vi "Motor Manager.vi"() -> ()   [LabVIEW 2014]
uses:
  Typedef/States - PC.ctl
  Typedef/Management variables.ctl
  LV Library/Typedef/Move type.ctl
  <vilib>/Instr/_visa.llb/VISA Configure Serial Port (Instr).vi
  LV Library/Motor manager.lvlib
panel:
  in  "Tab":enum32{"Manual movement", "Cycle"}(tab)
  in  "Down Button":bool
  in  "Up Button":bool
  in  "Right Button":bool
  in  "Left Button":bool
  in  "Speed":cluster{"Speed X":sgl, "Speed Y":sgl}={"Speed X"=10.0, "Speed Y"=10.0}
  in  "Acceleration":T1={"Acceleration X"=10, "Acceleration Y"=10}
  in  "Move type":enum32{"Absolute", "Step", "Free"}(radio)
  in  "Step":cluster{"Step X":sgl, "Step Y":sgl}={"Step X"=200.0, "Step Y"=200.0}
  in  "Cycle settings":T2
  in  "Stop process":bool
  in  "Keep torque":bool
  in  "Make Home":bool
  in  "Find Home":bool
  out "Connected?":bool
  in  "Connect":bool
  in  "VISA in":refnum<visa-resource-name>
  in  "Exit":bool
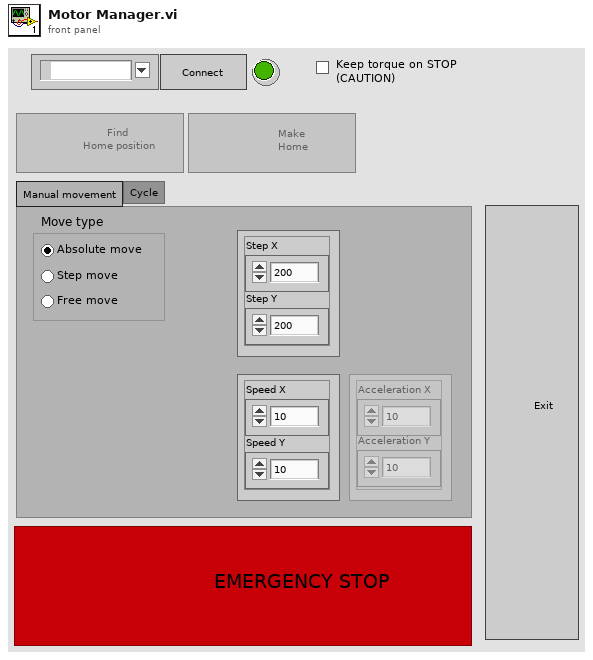
[diagram p1: front panel]
types:
  T1 = cluster{"Acceleration X":i32, "Acceleration Y":i32}
  T2 = cluster{"Motor":u8, "Distance":i32, "Speed":sgl, "IM delay":i32, "Cycle type":enum16{"Move forward first", "Move backward first"}, "N cycles":i32, "Go cycle":bool}
  T3 = typedef "Management variables.ctl" = cluster{"Keep torque":bool}
  T4 = typedef "States - PC.ctl" = enum16{"Connect", "Set speed", "Set management var", "Find Home", "Make Home", "Free Move up", "Free Move down", "Free Move right", "Free Move left", "Stop", "Step Move up", "Step Move down", "Step Move right", "Step Move left", "Simple Cycle", "Stop process", "Exit"}
  T5 = typedef "Motor manager.lvlib/Move type.ctl" = enum16{"Move forward", "Move backward", "Cycle (forward first)", "Cycle (backward first)", "Move step forward", "Move step backward"}
  T6 = cluster{T4, "Step":cluster{"Step X":sgl, "Step Y":sgl}}
  T7 = cluster{T4, "Cycle settings":cluster{"Motor":u8, "Distance":i32, "Speed":sgl, "IM delay":i32, "Cycle type":enum16{"Move forward first", "Move backward first"}, "N cycles":i32, "Go cycle":bool}}
  T8 = cluster{T4, "Speed":cluster{"Speed X":sgl, "Speed Y":sgl}}
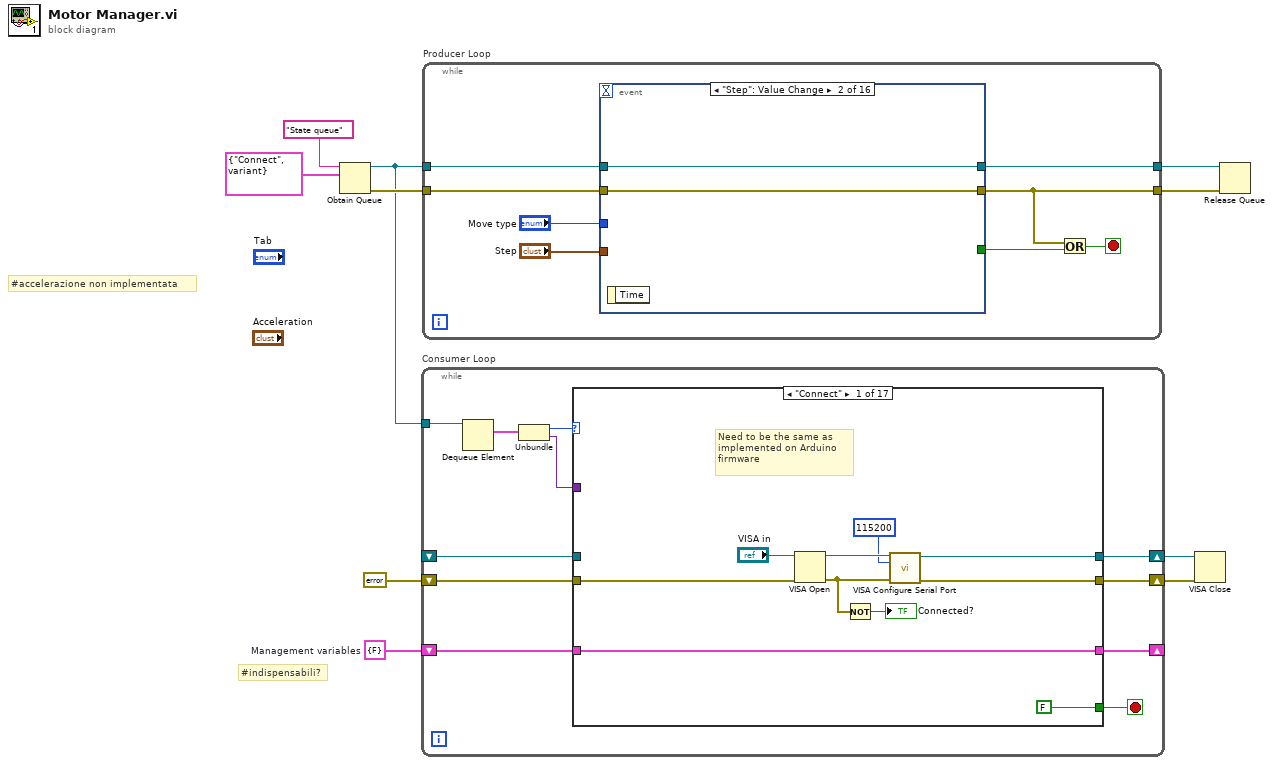
[diagram p0: block diagram]
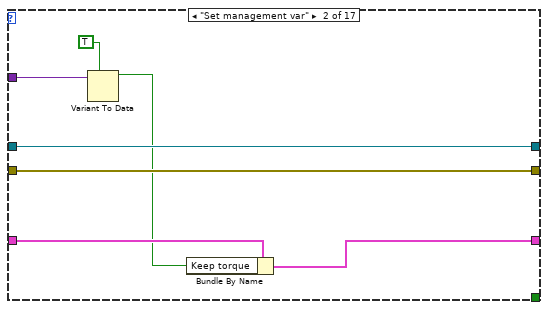
[diagram p2: hidden frame]
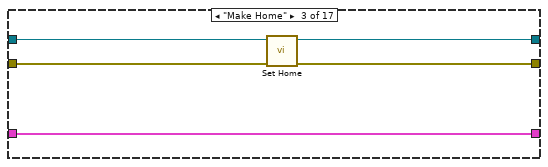
[diagram p3: hidden frame]
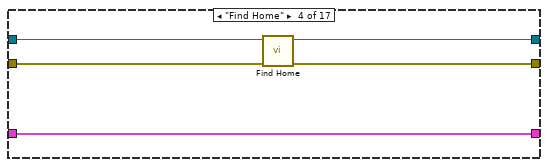
[diagram p4: hidden frame]
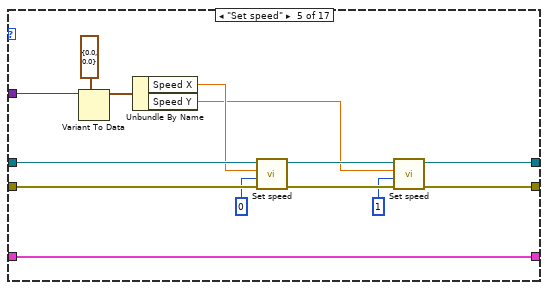
[diagram p5: hidden frame]
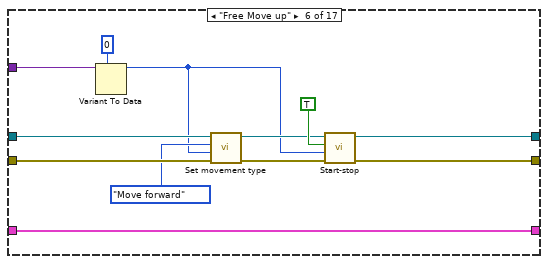
[diagram p6: hidden frame]
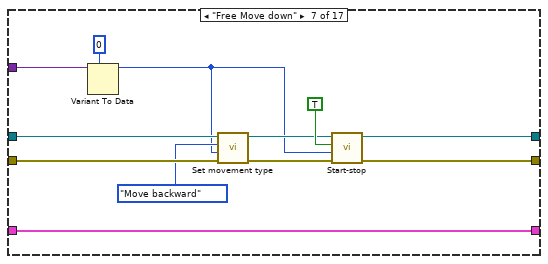
[diagram p7: hidden frame]
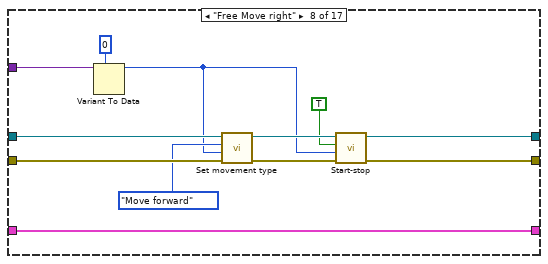
[diagram p8: hidden frame]
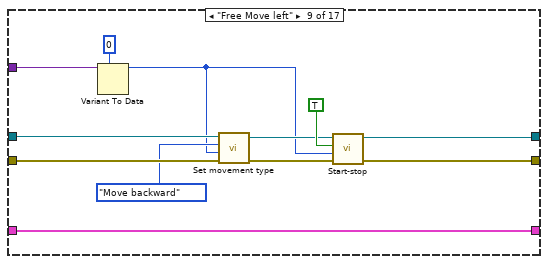
[diagram p9: hidden frame]
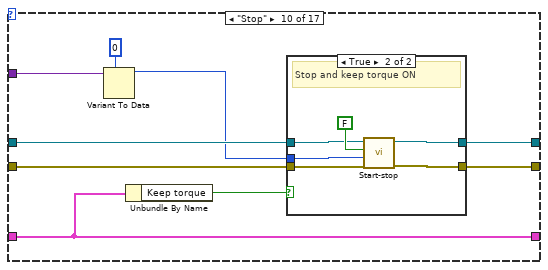
[diagram p10: hidden frame]
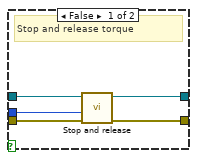
[diagram p11: hidden frame]
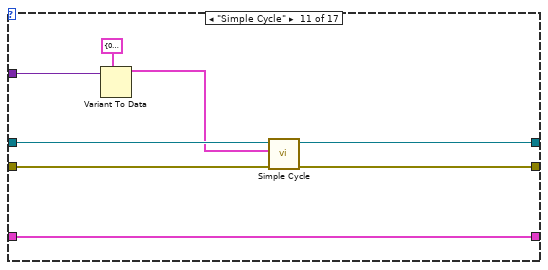
[diagram p12: hidden frame]
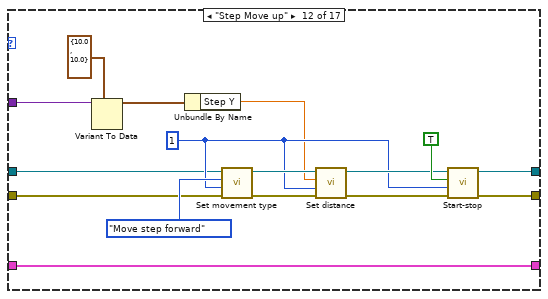
[diagram p13: hidden frame]
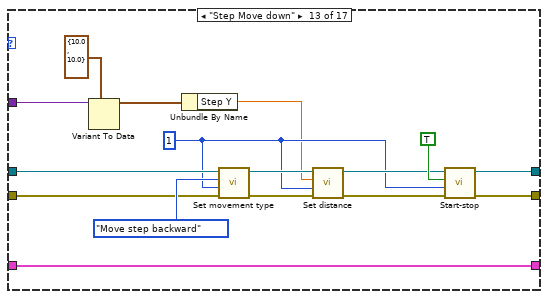
[diagram p14: hidden frame]
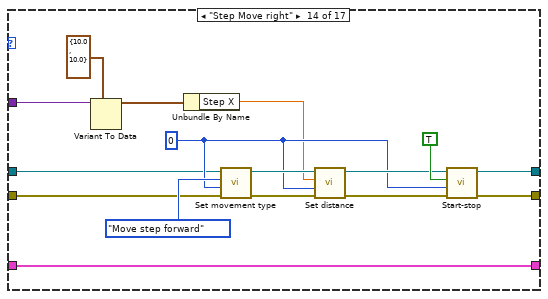
[diagram p15: hidden frame]
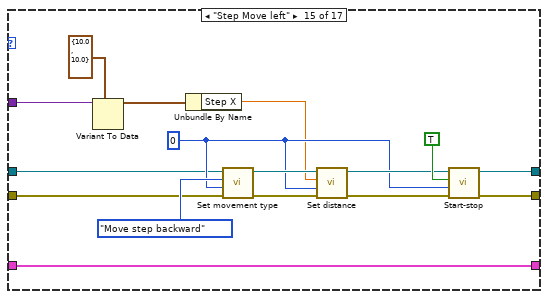
[diagram p16: hidden frame]
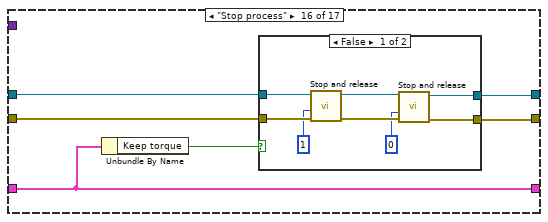
[diagram p17: hidden frame]
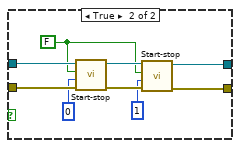
[diagram p18: hidden frame]
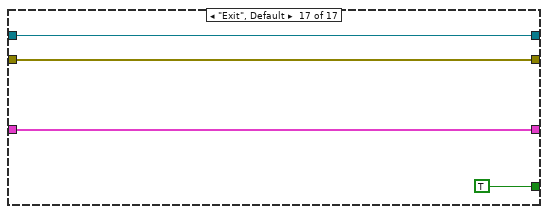
[diagram p19: hidden frame]
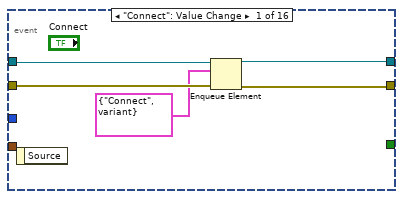
[diagram p20: hidden frame]
diagram:
  w2 = T3 {"Keep torque"=FALSE}  # Management variables
  # "#accelerazione non implementata"
  # "#indispensabili?"
  n1 = Obtain Queue(name (unnamed)="State queue", element data type=cluster{T4, variant} {enum."Connect", variant}) -> (queue out=w6:refnum<queue>, error out=w10:errorcluster)  [unwired: 3 in, 1 out]
  n2 = while "Consumer Loop" {
    tunnel: w6 -> [w21]
    shift-right: [w19] -> w5
    shift-left: _ -> [w17]
    shift-right: [w18] -> w4
    shift-left: errorcluster {"status"=FALSE, "code"=0, "source"=""} ("Error Out") -> [w16]
    shift-right: [w11] -> _
    shift-left: w2 -> [w12]
    stop <- w20 stop-if-true
    n3 = Dequeue Element(queue=w21) -> (element=w15:cluster{T4, variant})  [unwired: 2 in, 3 out]
    n4 = Unbundle(w15) -> (w14:T4, w13:variant)
    n5 = case shown="\"Connect\"" w14 {
      tunnel: [FALSE _ _ _ _ _ _ _ _ _ _ _ _ _ _ _ TRUE] -> w20
      tunnel: [w27 w38 w41 w45 w59 w73 w81 w93 w105 w118 w136 w140 w163 w173 w189 w206 w227] -> w19
      tunnel: [w26 w37 w39 w44 w60 w72 w80 w92 w104 w119 w135 w141 w164 w172 w188 w205 w226] -> w18
      tunnel: w17 -> [_ w38 w42 w46 w57 w70 w83 w94 w106 w117 w137 w143 w167 w175 w191 w208 w227]
      tunnel: w16 -> [w25 w37 w40 w47 w62 w71 w82 w95 w107 w116 w134 w142 w166 w176 w190 w207 w226]
      tunnel: w13 -> [_ w36 _ _ w56 w65 w78 w89 w101 w115 w132 w144 w168 w174 w192 _ _]
      tunnel: w12 -> [w22 w34 w43 w48 w49 w63 w75 w87 w99 w111 w138 w139 w165 w171 w187 w203 w228]
      tunnel: [w22 w32 w43 w48 w49 w63 w75 w87 w99 w111 w138 w139 w165 w171 w187 w203 w228] -> w11
      frame "Connect" {
        # "Need to be the same as \nimplemented on Arduino\nfirmware"
        n6 = VISA Open(error in (no error)=w25, VISA resource name="VISA in") -> (VISA resource name=w29:refnum<visa-resource-name>, error out=w24:errorcluster)  [unwired: 3 in]
        n7 = Not(x=w24) -> (.not. x?=→"Connected?":bool)
        n8 = call-poly "VISA Configure Serial Port"("VISA resource name"=w29, "baud rate (9600)"=u32 115200, "error in (no error)"=w24) -> ("VISA resource name out"=w27:refnum<visa-resource-name>, "error out"=w26:errorcluster)  [unwired: 11 in]
      }
      frame "Set management var" {
        n9 = Variant To Data(type=TRUE, Variant=w36) -> (data=w33:bool)  [unwired: 1 in, 1 out]
        n10 = Bundle By Name(cluster=w34, "Keep torque"=w33) -> (w32:T3)
      }
      frame "Make Home" {
        n11 = call "Set Home.vi"("Error In"=w40, "VISA resource in"=w42) -> ("Error Out"=w39:errorcluster, "VISA resource out"=w41:refnum<visa-resource-name>)  [unwired: 8 in]
      }
      frame "Find Home" {
        n12 = call "Find Home.vi"("Error In"=w47, "VISA resource in"=w46) -> ("Error Out"=w44:errorcluster, "VISA resource out"=w45:refnum<visa-resource-name>)  [unwired: 8 in]
      }
      frame "Set speed" {
        n13 = Variant To Data(type=cluster{"Speed X":sgl, "Speed Y":sgl} {"Speed X"=0.0, "Speed Y"=0.0} ("Speed 2"), Variant=w56) -> (data=w54:cluster{"Speed X":sgl, "Speed Y":sgl})  [unwired: 1 in, 1 out]
        n14 = Unbundle By Name(w54) -> ("Speed X"=w53:sgl, "Speed Y"=w52:sgl)
        n15 = call "Set speed.vi"("Error In"=w62, "Motor index"=u8 0, "Speed"=w53, "VISA resource in"=w57) -> ("Error Out"=w61:errorcluster, "VISA resource out"=w58:refnum<visa-resource-name>)  [unwired: 6 in]
        n16 = call "Set speed.vi"("Error In"=w61, "Motor index"=u8 1, "Speed"=w52, "VISA resource in"=w58) -> ("Error Out"=w60:errorcluster, "VISA resource out"=w59:refnum<visa-resource-name>)  [unwired: 6 in]
      }
      frame "Free Move up" {
        n17 = Variant To Data(type=u8 0, Variant=w65) -> (data=w64:u8)  [unwired: 1 in, 1 out]
        n18 = call "Set movement type.vi"("Error In"=w71, "Motor index"=w64, "Movement type"=Move_type."Move forward", "VISA resource in"=w70) -> ("Error Out"=w69:errorcluster, "VISA resource out"=w68:refnum<visa-resource-name>)  [unwired: 6 in]
        n19 = call "Start-stop.vi"("Error In"=w69, "Motor index"=w64, "Go"=TRUE, "VISA resource in"=w68) -> ("Error Out"=w72:errorcluster, "VISA resource out"=w73:refnum<visa-resource-name>)  [unwired: 6 in]
      }
      frame "Free Move down" {
        n20 = Variant To Data(type=u8 0, Variant=w78) -> (data=w76:u8)  [unwired: 1 in, 1 out]
        n21 = call "Set movement type.vi"("Error In"=w82, "Motor index"=w76, "Movement type"=Move_type."Move backward", "VISA resource in"=w83) -> ("Error Out"=w85:errorcluster, "VISA resource out"=w84:refnum<visa-resource-name>)  [unwired: 6 in]
        n22 = call "Start-stop.vi"("Error In"=w85, "Motor index"=w76, "Go"=TRUE, "VISA resource in"=w84) -> ("Error Out"=w80:errorcluster, "VISA resource out"=w81:refnum<visa-resource-name>)  [unwired: 6 in]
      }
      frame "Free Move right" {
        n23 = Variant To Data(type=u8 0, Variant=w89) -> (data=w88:u8)  [unwired: 1 in, 1 out]
        n24 = call "Set movement type.vi"("Error In"=w95, "Motor index"=w88, "Movement type"=Move_type."Move forward", "VISA resource in"=w94) -> ("Error Out"=w97:errorcluster, "VISA resource out"=w98:refnum<visa-resource-name>)  [unwired: 6 in]
        n25 = call "Start-stop.vi"("Error In"=w97, "Motor index"=w88, "Go"=TRUE, "VISA resource in"=w98) -> ("Error Out"=w92:errorcluster, "VISA resource out"=w93:refnum<visa-resource-name>)  [unwired: 6 in]
      }
      frame "Free Move left" {
        n26 = Variant To Data(type=u8 0, Variant=w101) -> (data=w100:u8)  [unwired: 1 in, 1 out]
        n27 = call "Set movement type.vi"("Error In"=w107, "Motor index"=w100, "Movement type"=Move_type."Move backward", "VISA resource in"=w106) -> ("Error Out"=w109:errorcluster, "VISA resource out"=w108:refnum<visa-resource-name>)  [unwired: 6 in]
        n28 = call "Start-stop.vi"("Error In"=w109, "Motor index"=w100, "Go"=TRUE, "VISA resource in"=w108) -> ("Error Out"=w104:errorcluster, "VISA resource out"=w105:refnum<visa-resource-name>)  [unwired: 6 in]
      }
      frame "Stop" {
        n29 = Variant To Data(type=u8 0, Variant=w115) -> (data=w113:u8)  [unwired: 1 in, 1 out]
        n30 = Unbundle By Name(w111) -> ("Keep torque"=w112:bool)
        n31 = case shown="True" w112 {
          tunnel: [w120 w129] -> w119
          tunnel: [w123 w128] -> w118
          tunnel: w117 -> [w124 w127]
          tunnel: w116 -> [w122 w126]
          tunnel: w113 -> [w121 w125]
          frame False {
            # "Stop and release torque"
            n32 = call "Stop and release.vi"("Error In"=w122, "Motor index"=w121, "VISA resource in"=w124) -> ("Error Out"=w120:errorcluster, "VISA resource out"=w123:refnum<visa-resource-name>)  [unwired: 7 in]
          }
          frame True {
            # "Stop and keep torque ON"
            n33 = call "Start-stop.vi"("Error In"=w126, "Motor index"=w125, "Go"=FALSE, "VISA resource in"=w127) -> ("Error Out"=w129:errorcluster, "VISA resource out"=w128:refnum<visa-resource-name>)  [unwired: 6 in]
          }
        }
      }
      frame "Simple Cycle" {
        n34 = Variant To Data(type=T2 {"Motor"=0, "Distance"=0, "Speed"=0.0, "IM delay"=0, "Cycle type"=enum."Move forward first", "N cycles"=0, "Go cycle"=FALSE} ("Cycle settings 2"), Variant=w132) -> (data=w131:T2)  [unwired: 1 in, 1 out]
        n35 = call "Simple Cycle.vi"("Error In"=w134, "Cycle settings"=w131, "VISA in"=w137) -> ("Error Out"=w135:errorcluster, "VISA out"=w136:refnum<visa-resource-name>)  [unwired: 7 in]
      }
      frame "Step Move up" {
        w147 = u8 1
        n36 = Variant To Data(type=cluster{"Step X":sgl, "Step Y":sgl} {"Step X"=10.0, "Step Y"=10.0} ("Step"), Variant=w144) -> (data=w146:cluster{"Step X":sgl, "Step Y":sgl})  [unwired: 1 in, 1 out]
        n37 = Unbundle By Name(w146) -> ("Step Y"=w145:sgl)
        n38 = call "Set movement type.vi"("Error In"=w142, "Motor index"=w147, "Movement type"=Move_type."Move step forward", "VISA resource in"=w143) -> ("Error Out"=w151:errorcluster, "VISA resource out"=w152:refnum<visa-resource-name>)  [unwired: 6 in]
        n39 = call "Set distance.vi"("Error In"=w151, "Motor index"=w147, "Travel distance"=w145, "VISA resource in"=w152) -> ("Error Out"=w150:errorcluster, "VISA resource out"=w149:refnum<visa-resource-name>)  [unwired: 6 in]
        n40 = call "Start-stop.vi"("Error In"=w150, "Motor index"=w147, "Go"=TRUE, "VISA resource in"=w149) -> ("Error Out"=w141:errorcluster, "VISA resource out"=w140:refnum<visa-resource-name>)  [unwired: 6 in]
      }
      frame "Step Move down" {
        w157 = u8 1
        n41 = Variant To Data(type=cluster{"Step X":sgl, "Step Y":sgl} {"Step X"=10.0, "Step Y"=10.0} ("Step"), Variant=w168) -> (data=w156:cluster{"Step X":sgl, "Step Y":sgl})  [unwired: 1 in, 1 out]
        n42 = Unbundle By Name(w156) -> ("Step Y"=w155:sgl)
        n43 = call "Set movement type.vi"("Error In"=w166, "Motor index"=w157, "Movement type"=Move_type."Move step backward", "VISA resource in"=w167) -> ("Error Out"=w161:errorcluster, "VISA resource out"=w162:refnum<visa-resource-name>)  [unwired: 6 in]
        n44 = call "Set distance.vi"("Error In"=w161, "Motor index"=w157, "Travel distance"=w155, "VISA resource in"=w162) -> ("Error Out"=w160:errorcluster, "VISA resource out"=w159:refnum<visa-resource-name>)  [unwired: 6 in]
        n45 = call "Start-stop.vi"("Error In"=w160, "Motor index"=w157, "Go"=TRUE, "VISA resource in"=w159) -> ("Error Out"=w164:errorcluster, "VISA resource out"=w163:refnum<visa-resource-name>)  [unwired: 6 in]
      }
      frame "Step Move right" {
        w179 = u8 0
        n46 = Variant To Data(type=cluster{"Step X":sgl, "Step Y":sgl} {"Step X"=10.0, "Step Y"=10.0} ("Step"), Variant=w174) -> (data=w178:cluster{"Step X":sgl, "Step Y":sgl})  [unwired: 1 in, 1 out]
        n47 = Unbundle By Name(w178) -> ("Step X"=w177:sgl)
        n48 = call "Set movement type.vi"("Error In"=w176, "Motor index"=w179, "Movement type"=Move_type."Move step forward", "VISA resource in"=w175) -> ("Error Out"=w183:errorcluster, "VISA resource out"=w184:refnum<visa-resource-name>)  [unwired: 6 in]
        n49 = call "Set distance.vi"("Error In"=w183, "Motor index"=w179, "Travel distance"=w177, "VISA resource in"=w184) -> ("Error Out"=w182:errorcluster, "VISA resource out"=w181:refnum<visa-resource-name>)  [unwired: 6 in]
        n50 = call "Start-stop.vi"("Error In"=w182, "Motor index"=w179, "Go"=TRUE, "VISA resource in"=w181) -> ("Error Out"=w172:errorcluster, "VISA resource out"=w173:refnum<visa-resource-name>)  [unwired: 6 in]
      }
      frame "Step Move left" {
        w195 = u8 0
        n51 = Variant To Data(type=cluster{"Step X":sgl, "Step Y":sgl} {"Step X"=10.0, "Step Y"=10.0} ("Step"), Variant=w192) -> (data=w194:cluster{"Step X":sgl, "Step Y":sgl})  [unwired: 1 in, 1 out]
        n52 = Unbundle By Name(w194) -> ("Step X"=w193:sgl)
        n53 = call "Set movement type.vi"("Error In"=w190, "Motor index"=w195, "Movement type"=Move_type."Move step backward", "VISA resource in"=w191) -> ("Error Out"=w199:errorcluster, "VISA resource out"=w200:refnum<visa-resource-name>)  [unwired: 6 in]
        n54 = call "Set distance.vi"("Error In"=w199, "Motor index"=w195, "Travel distance"=w193, "VISA resource in"=w200) -> ("Error Out"=w198:errorcluster, "VISA resource out"=w197:refnum<visa-resource-name>)  [unwired: 6 in]
        n55 = call "Start-stop.vi"("Error In"=w198, "Motor index"=w195, "Go"=TRUE, "VISA resource in"=w197) -> ("Error Out"=w188:errorcluster, "VISA resource out"=w189:refnum<visa-resource-name>)  [unwired: 6 in]
      }
      frame "Stop process" {
        n56 = Unbundle By Name(w203) -> ("Keep torque"=w204:bool)
        n57 = case shown="False" w204 {
          tunnel: w208 -> [w215 w223]
          tunnel: w207 -> [w216 w222]
          tunnel: [w211 w221] -> w206
          tunnel: [w212 w220] -> w205
          frame False {
            n58 = call "Stop and release.vi"("Error In"=w216, "Motor index"=u8 1, "VISA resource in"=w215) -> ("Error Out"=w213:errorcluster, "VISA resource out"=w214:refnum<visa-resource-name>)  [unwired: 7 in]
            n59 = call "Stop and release.vi"("Error In"=w213, "Motor index"=u8 0, "VISA resource in"=w214) -> ("Error Out"=w212:errorcluster, "VISA resource out"=w211:refnum<visa-resource-name>)  [unwired: 7 in]
          }
          frame True {
            w217 = FALSE ("Go")
            n60 = call "Start-stop.vi"("Error In"=w222, "Motor index"=u8 0, "Go"=w217, "VISA resource in"=w223) -> ("Error Out"=w224:errorcluster, "VISA resource out"=w225:refnum<visa-resource-name>)  [unwired: 6 in]
            n61 = call "Start-stop.vi"("Error In"=w224, "Motor index"=u8 1, "Go"=w217, "VISA resource in"=w225) -> ("Error Out"=w220:errorcluster, "VISA resource out"=w221:refnum<visa-resource-name>)  [unwired: 6 in]
          }
        }
      }
      frame "Exit", Default {
      }
    }
  }
  n62 = while "Producer Loop" {
    tunnel: w6 -> [w237]
    tunnel: w10 -> [w236]
    tunnel: [w232] -> w8
    tunnel: [w235] -> w7
    stop <- w234 stop-if-true
    n63 = event shown="[1] \"Step\": Value Change" {
      selector: _ -> [_ _ _ _ _ _ _ _ _ _ _ _ _ _ _ _]
      dyn-events: _ -> [_ _ _ _ _ _ _ _ _ _ _ _ _ _ _ _]
      timeout: _ -> [_ _ _ _ _ _ _ _ _ _ _ _ _ _ _ _]
      tunnel: w237 -> [w241 w244 w248 w252 w258 w277 w299 w315 w319 w338 w358 w371 w377 w384 w391 w394]
      tunnel: w236 -> [w242 w243 w249 w251 w257 w278 w298 w314 w318 w337 w357 w370 w378 w383 w390 w395]
      tunnel: [w239 w244 w247 w254 w259 w280 w297 w312 w321 w341 w360 w371 w376 w382 w389 w393] -> w235
      tunnel: [w240 w243 w246 w253 w260 w279 w296 w313 w320 w340 w359 w370 w375 w381 w388 w392] -> w232
      tunnel: [_ _ _ _ _ _ _ _ _ _ _ _ _ TRUE _ _] -> w233
      tunnel: "Move type" -> [_ _ _ _ w256 w276 w295 _ w316 w336 w356 _ _ _ _ _]
      tunnel: "Step" -> [_ _ _ _ w255 w275 _ _ w317 w339 _ _ _ _ _ _]
      event "Connect": Value Change {
        n64 = event-data() -> ()  [unwired: 1 in, 1 out]
        n65 = Enqueue Element(queue=w241, element=cluster{T4, variant} {enum."Connect", variant}, error in (no error)=w242) -> (queue out=w239:refnum<queue>, error out=w240:errorcluster)  [unwired: 1 in, 1 out]
      }
      event "Step": Value Change {
        n66 = event-data() -> ()  [unwired: 1 in, 1 out]
      }
      event "Find Home": Value Change {
        n67 = event-data() -> ()  [unwired: 1 in, 1 out]
        n68 = Enqueue Element(queue=w248, element=cluster{T4, variant} {enum."Find Home", variant}, error in (no error)=w249) -> (queue out=w247:refnum<queue>, error out=w246:errorcluster)  [unwired: 1 in, 1 out]
      }
      event "Make Home": Value Change {
        n69 = event-data() -> ()  [unwired: 1 in, 1 out]
        n70 = Enqueue Element(queue=w252, element=cluster{T4, variant} {enum."Make Home", variant}, error in (no error)=w251) -> (queue out=w254:refnum<queue>, error out=w253:errorcluster)  [unwired: 1 in, 1 out]
      }
      event "Up Button": Mouse Down {
        n71 = event-data() -> ()  [unwired: 1 in, 1 out]
        n72 = case shown="\"Free\", Default" w256 {
          tunnel: [w265 w267 w272] -> w259
          tunnel: [w264 w266 w271] -> w260
          tunnel: w257 -> [w263 w266 w274]
          tunnel: w258 -> [w262 w267 w273]
          tunnel: w255 -> [_ _ w269]
          frame "Free", Default {
            n73 = Enqueue Element(queue=w262, element=cluster{T4, i32} {enum."Free Move up", 1}, error in (no error)=w263) -> (queue out=w265:refnum<queue>, error out=w264:errorcluster)  [unwired: 1 in, 1 out]
          }
          frame "Absolute" {
            # "#notImplemented"
          }
          frame "Step" {
            n74 = Bundle(States_-_PC."Step Move up", "Step"=w269) -> (w268:T6)  [unwired: 1 in]
            n75 = Enqueue Element(queue=w273, element=w268, error in (no error)=w274) -> (queue out=w272:refnum<queue>, error out=w271:errorcluster)  [unwired: 1 in, 1 out]
          }
        }
      }
      event "Down Button": Mouse Down {
        n76 = event-data() -> ()  [unwired: 1 in, 1 out]
        n77 = case shown="\"Free\", Default" w276 {
          tunnel: [w285 w287 w292] -> w280
          tunnel: [w284 w286 w291] -> w279
          tunnel: w278 -> [w283 w286 w294]
          tunnel: w277 -> [w282 w287 w293]
          tunnel: w275 -> [_ _ w289]
          frame "Free", Default {
            n78 = Enqueue Element(queue=w282, element=cluster{T4, i32} {enum."Free Move down", 1}, error in (no error)=w283) -> (queue out=w285:refnum<queue>, error out=w284:errorcluster)  [unwired: 1 in, 1 out]
          }
          frame "Absolute" {
            # "#notImplemented"
          }
          frame "Step" {
            n79 = Bundle(States_-_PC."Step Move down", "Step"=w289) -> (w288:T6)  [unwired: 1 in]
            n80 = Enqueue Element(queue=w293, element=w288, error in (no error)=w294) -> (queue out=w292:refnum<queue>, error out=w291:errorcluster)  [unwired: 1 in, 1 out]
          }
        }
      }
      event "Up Button", "Down Button": Mouse Up {
        n81 = event-data() -> ()  [unwired: 1 in, 1 out]
        n82 = case shown="\"Step\"" w295 {
          tunnel: w299 -> [w301 w303 w308]
          tunnel: w298 -> [w300 w302 w307]
          tunnel: [w301 w303 w306] -> w297
          tunnel: [w300 w302 w305] -> w296
          frame "Absolute", Default {
          }
          frame "Step" {
          }
          frame "Free" {
            n83 = Enqueue Element(queue=w308, element=cluster{T4, u8} {enum."Stop", 1}, error in (no error)=w307) -> (queue out=w306:refnum<queue>, error out=w305:errorcluster)  [unwired: 1 in, 1 out]
          }
        }
      }
      event "Cycle settings.Go cycle": Value Change {
        n84 = event-data() -> ()  [unwired: 1 in, 1 out]
        n85 = Bundle(States_-_PC."Simple Cycle", "Cycle settings"="Cycle settings") -> (w309:T7)  [unwired: 1 in]
        n86 = Enqueue Element(queue=w315, element=w309, error in (no error)=w314) -> (queue out=w312:refnum<queue>, error out=w313:errorcluster)  [unwired: 1 in, 1 out]
      }
      event "Right Button": Mouse Down {
        n87 = event-data() -> ()  [unwired: 1 in, 1 out]
        n88 = case shown="\"Free\", Default" w316 {
          tunnel: [w326 w328 w333] -> w321
          tunnel: [w325 w327 w332] -> w320
          tunnel: w318 -> [w324 w327 w335]
          tunnel: w319 -> [w323 w328 w334]
          tunnel: w317 -> [_ _ w330]
          frame "Free", Default {
            n89 = Enqueue Element(queue=w323, element=cluster{T4, i32} {enum."Free Move right", 0}, error in (no error)=w324) -> (queue out=w326:refnum<queue>, error out=w325:errorcluster)  [unwired: 1 in, 1 out]
          }
          frame "Absolute" {
            # "#notImplemented"
          }
          frame "Step" {
            n90 = Bundle(States_-_PC."Step Move right", "Step"=w330) -> (w329:T6)  [unwired: 1 in]
            n91 = Enqueue Element(queue=w334, element=w329, error in (no error)=w335) -> (queue out=w333:refnum<queue>, error out=w332:errorcluster)  [unwired: 1 in, 1 out]
          }
        }
      }
      event "Left Button": Mouse Down {
        n92 = event-data() -> ()  [unwired: 1 in, 1 out]
        n93 = case shown="\"Free\", Default" w336 {
          tunnel: [w346 w348 w353] -> w341
          tunnel: [w345 w347 w352] -> w340
          tunnel: w337 -> [w344 w347 w355]
          tunnel: w338 -> [w343 w348 w354]
          tunnel: w339 -> [_ _ w350]
          frame "Free", Default {
            n94 = Enqueue Element(queue=w343, element=cluster{T4, i32} {enum."Free Move left", 0}, error in (no error)=w344) -> (queue out=w346:refnum<queue>, error out=w345:errorcluster)  [unwired: 1 in, 1 out]
          }
          frame "Absolute" {
            # "#notImplemented"
          }
          frame "Step" {
            n95 = Bundle(States_-_PC."Step Move left", "Step"=w350) -> (w349:T6)  [unwired: 1 in]
            n96 = Enqueue Element(queue=w354, element=w349, error in (no error)=w355) -> (queue out=w353:refnum<queue>, error out=w352:errorcluster)  [unwired: 1 in, 1 out]
          }
        }
      }
      event "Left Button", "Right Button": Mouse Up {
        n97 = event-data() -> ()  [unwired: 1 in, 1 out]
        n98 = case shown="\"Step\"" w356 {
          tunnel: [w362 w364 w369] -> w360
          tunnel: [w361 w363 w368] -> w359
          tunnel: w358 -> [w362 w364 w367]
          tunnel: w357 -> [w361 w363 w366]
          frame "Absolute", Default {
          }
          frame "Step" {
          }
          frame "Free" {
            n99 = Enqueue Element(queue=w367, element=cluster{T4, u8} {enum."Stop", 0}, error in (no error)=w366) -> (queue out=w369:refnum<queue>, error out=w368:errorcluster)  [unwired: 1 in, 1 out]
          }
        }
      }
      event "Move type": Value Change {
        n100 = event-data() -> ()  [unwired: 1 in, 1 out]
      }
      event "Speed": Value Change {
        n101 = event-data() -> ()  [unwired: 1 in, 6 out]
        n102 = Bundle(States_-_PC."Set speed", "Speed"="Speed") -> (w372:T8)  [unwired: 1 in]
        n103 = Enqueue Element(queue=w377, element=w372, error in (no error)=w378) -> (queue out=w376:refnum<queue>, error out=w375:errorcluster)  [unwired: 1 in, 1 out]
      }
      event "Exit": Value Change {
        n104 = event-data() -> ()  [unwired: 1 in, 1 out]
        n105 = Enqueue Element(queue=w384, element=cluster{T4, variant} {enum."Exit", variant}, error in (no error)=w383) -> (queue out=w382:refnum<queue>, error out=w381:errorcluster)  [unwired: 1 in, 1 out]
      }
      event "Keep torque": Value Change {
        n106 = event-data() -> ("NewVal"=w386:bool)  [unwired: 1 in]
        n107 = Bundle(States_-_PC."Set management var", "NewVal"=w386) -> (w385:cluster{T4, "NewVal":bool})  [unwired: 1 in]
        n108 = Enqueue Element(queue=w391, element=w385, error in (no error)=w390) -> (queue out=w389:refnum<queue>, error out=w388:errorcluster)  [unwired: 1 in, 1 out]
      }
      event "Stop process": Value Change {
        n109 = event-data() -> ()  [unwired: 1 in, 2 out]
        n110 = Enqueue Element(queue=w394, element=cluster{T4, bool} {enum."Stop process", FALSE}, error in (no error)=w395) -> (queue out=w393:refnum<queue>, error out=w392:errorcluster)  [unwired: 1 in, 1 out]
      }
    }
    n111 = Or(x=w232, y=w233) -> (x .or. y?=w234:bool)
  }
  n112 = VISA Close(VISA resource name=w5, error in (no error)=w4) -> ()  [unwired: 1 out]
  n113 = Release Queue(queue=w7, error in (no error)=w8) -> ()  [unwired: 1 in, 3 out]
